vi "HEWH Specific Message.vi"(8 "Error In":errorcluster, 10 "Message Adder":string, 11 "element":T1={"Sequence #"=0.0, "Cycles"=0, "Mode Setting"="", "Flow Rate (GPM)"=0.0, "Temperature (F)"=0.0, "Reset Timer"=FALSE, "Use Temp Decline Method"=FALSE, "Terminate Condition"=enum."C1-Terminate Draw @ Gallon Mark", "Condition Value #1"=0.0, "UE"=FALSE, "LE"=FALSE, "Comp"=FALSE, "Fan"=FALSE, "Test End Time (Sec)"=0.0, "Purge Until Cutout"=FALSE, "Start Conditions"=enum."Heat Source Cutout", "Condition Value #2"=0.0, "Remove Power"=FALSE, "Time"=0.0, "Check Special Cond."=enum."SC1-Do Nothing", "Condition#"=enum."C1", "Draw Flags"=enum."N/A", "Data Processing Delay (FHD 15sec, UEF 5 Sec)"=0.0, "Test Complete"=FALSE} {"Time" format="%<%H:%M:%S>t"}) -> (0 "Error Out":errorcluster, 3 "Message":string)   [LabVIEW 2016]
uses:
  Type Definitions/PRAT Test.ctl
  Utility/Save File/File Setup (Public)/Type Definition/Save File HEWH Heating Control Mode.ctl
  Type Definitions/Terminate Draw Conditions.ctl
  Type Definitions/HEWH Start Conditions.ctl
  Type Definitions/Check Special Condtions.ctl
  Type Definitions/HEWH Special Condition Check.ctl
  Type Definitions/HEWH Draw Flag ENUM.ctl
  <vilib>/Utility/error.llb/whitespace.ctl
  Utility/Save File/File Setup.lvlib
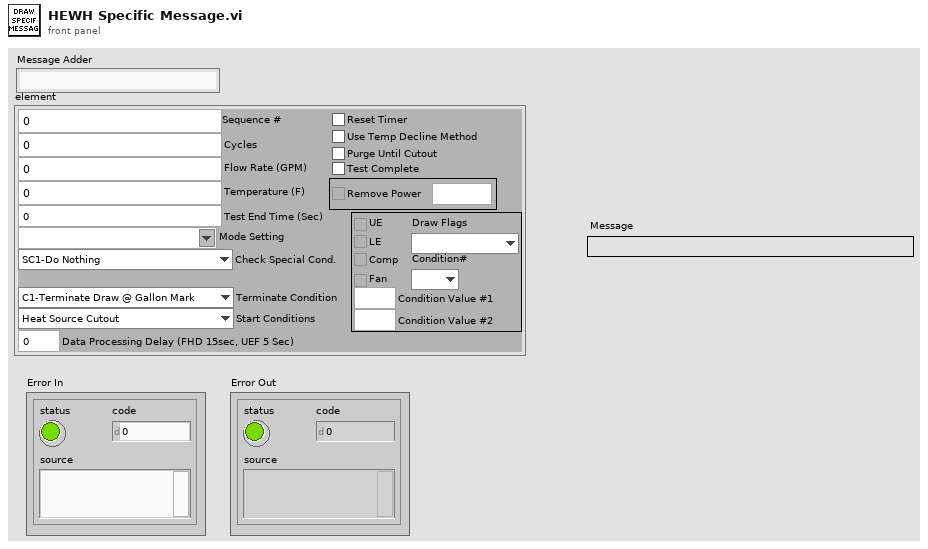
[diagram p1: front panel]
types:
  T1 = typedef "PRAT Test.ctl" = cluster{"Sequence #":dbl, "Cycles":i32, "Mode Setting":T2, "Flow Rate (GPM)":dbl, "Temperature (F)":dbl, "Reset Timer":bool, "Use Temp Decline Method":bool, "Terminate Condition":T3, "Condition Value #1":dbl, "UE":bool, "LE":bool, "Comp":bool, "Fan":bool, "Test End Time (Sec)":dbl, "Purge Until Cutout":bool, "Start Conditions":T4, "Condition Value #2":dbl, "Remove Power":bool, "Time":dbl, "Check Special Cond.":T5, "Condition#":T6, "Draw Flags":T7, "Data Processing Delay (FHD 15sec, UEF 5 Sec)":dbl, "Test Complete":bool}
  T2 = typedef "File Setup.lvlib/Save File HEWH Heating Control Mode.ctl" = string
  T3 = typedef "Terminate Draw Conditions.ctl" = enum16{"C1-Terminate Draw @ Gallon Mark", "C2-Special Last Draw (HU Test)", "C3-RTD Out <=", "C4-Mean Tank Temp <=", "C5-Decrease RTD Out (Deg F)", "C6-Time (Seconds)", "C7-Until Any Heat Source", "C8-Specific Heat Source", "C9-Do Nothing"}
  T4 = typedef "HEWH Start Conditions.ctl" = enum16{"Heat Source Cutout", "At Time (Seconds)", "Every X (Seconds)", "T2 >= X° Below Setpoint", "Seconds From Complete", "Wait for LE & Comp Cutout", "Wait for Comp Cutout", "Wait for LE Cutout", "Wait for UE Cutout"}
  T5 = typedef "Check Special Condtions.ctl" = enum16{"SC1-Do Nothing", "SC2-Check Heat Source (On-C2/Off-C1)", "SC3-Check Skip Condition", "SC4-Check Heat Source ON/Fail"}
  T6 = typedef "HEWH Special Condition Check.ctl" = enum16{"N/A", "C1", "C2", "Reset/Fail", "Skip Draw Sequence"}
  T7 = typedef "HEWH Draw Flag ENUM.ctl" = enum16{"N/A", "None(0)", "Sml(1)", "Med(2)", "SmlMed(3)", "Lrg(4)", "SmlLrg(5)", "MedLrg(6)", "SmlMedLrg(7)"}
  T8 = typedef "whitespace.ctl" = u16
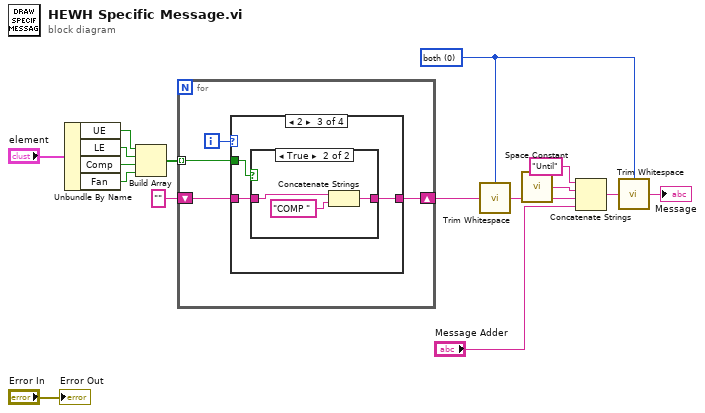
[diagram p0: block diagram]
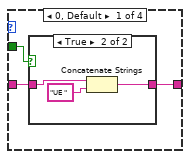
[diagram p2: hidden frame]
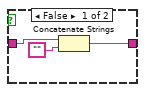
[diagram p3: hidden frame]
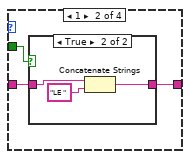
[diagram p4: hidden frame]
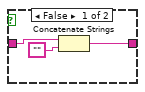
[diagram p5: hidden frame]
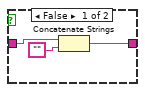
[diagram p6: hidden frame]
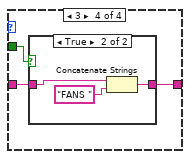
[diagram p7: hidden frame]
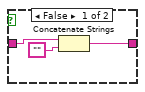
[diagram p8: hidden frame]
diagram:
  w1 = T8 0 items=["both", "start of string", "end of string"] ("location (both)")
  n1 = Unbundle By Name("element") -> ("UE"=w15:bool, "LE"=w14:bool, "Comp"=w13:bool, "Fan"=w12:bool)
  n2 = Build Array(w15, w14, w13, w12) -> (w11:bool[])
  n3 = for {
    shift-right: [w20] -> w10
    shift-left: "" -> [w19]
    tunnel: w11 -> [w17] mode=indexing
    i -> [w18]
    n4 = case shown="2" w18 {
      tunnel: [w22 w32 w41 w48] -> w20
      tunnel: w19 -> [w23 w31 w40 w49]
      tunnel: w17 -> [w21 w30 w39 w50]
      frame 0, Default {
        n5 = case shown="True" w21 {
          tunnel: [w26 w28] -> w22
          tunnel: w23 -> [w25 w29]
          frame False {
            n6 = Concatenate Strings(w25, "") -> (w26:string)
          }
          frame True {
            n7 = Concatenate Strings(w29, "UE " ("string")) -> (w28:string)
          }
        }
      }
      frame 1 {
        n8 = case shown="True" w30 {
          tunnel: [w35 w37] -> w32
          tunnel: w31 -> [w34 w38]
          frame False {
            n9 = Concatenate Strings(w34, "") -> (w35:string)
          }
          frame True {
            n10 = Concatenate Strings(w38, "LE " ("string")) -> (w37:string)
          }
        }
      }
      frame 2 {
        n11 = case shown="True" w39 {
          tunnel: [w44 w46] -> w41
          tunnel: w40 -> [w43 w47]
          frame False {
            n12 = Concatenate Strings(w43, "") -> (w44:string)
          }
          frame True {
            n13 = Concatenate Strings(w47, "COMP " ("string")) -> (w46:string)
          }
        }
      }
      frame 3 {
        n14 = case shown="True" w50 {
          tunnel: [w53 w55] -> w48
          tunnel: w49 -> [w52 w56]
          frame False {
            n15 = Concatenate Strings(w52, "") -> (w53:string)
          }
          frame True {
            n16 = Concatenate Strings(w56, "FANS " ("string")) -> (w55:string)
          }
        }
      }
    }
  }
  n17 = call <vilib>:"Trim Whitespace.vi"("string"=w10, "location (both)"=w1) -> ("trimmed string"=w9:string)
  n18 = call <vilib>:"Space Constant.vi"() -> ("String"=w7:string)
  n19 = Concatenate Strings("Until" ("string"), w7, w9, "Message Adder") -> (w3:string)
  n20 = call <vilib>:"Trim Whitespace.vi"("string"=w3, "location (both)"=w1) -> ("trimmed string"=→"Message":string)
  "Error Out" <- "Error In"
